vi "initialise.vi"(8 "error in (no error)":errorcluster, 11 "ScanHeadMH100729FPGA in":refnum<class "ScanHeadMH100729FPGA.lvclass">) -> (0 "error out":errorcluster, 3 "ScanHeadMH100729FPGA out":refnum<class "ScanHeadMH100729FPGA.lvclass">)   [LabVIEW 2010, in "ScanHeadMH100729FPGA.lvclass"]
uses:
  ScanHeadMH100729FPGA.lvclass
  GenericScanHead/GenericScanHead/GenericScanHead.lvclass
  ScanHeadMH100729FPGA.lvclass/ScanHeadMH100729FPGA.ctl
  AnalogOut/GenericAnalogOut/GenericAnalogOut/GenericAnalogOut.lvclass
  common/classes/ErrorController/ErrorController/class_data.vi
  common/classes/ErrorController/ErrorController/ErrorController.lvclass
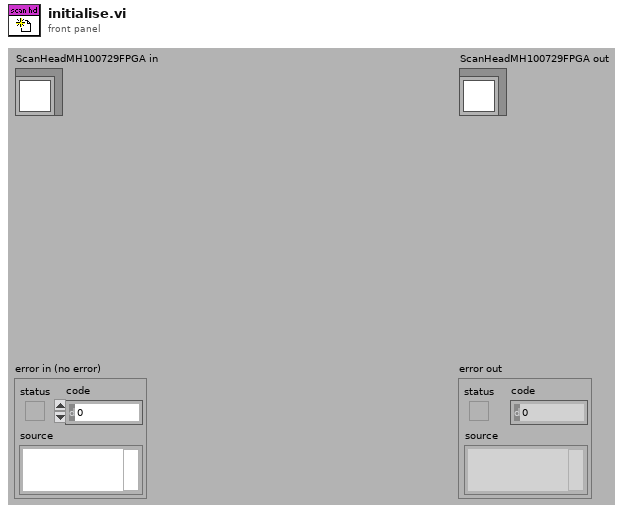
[diagram p1: front panel]
types:
  T1 = enum8{"Enabled", "Disabled", "Disabled and Grayed Out"}
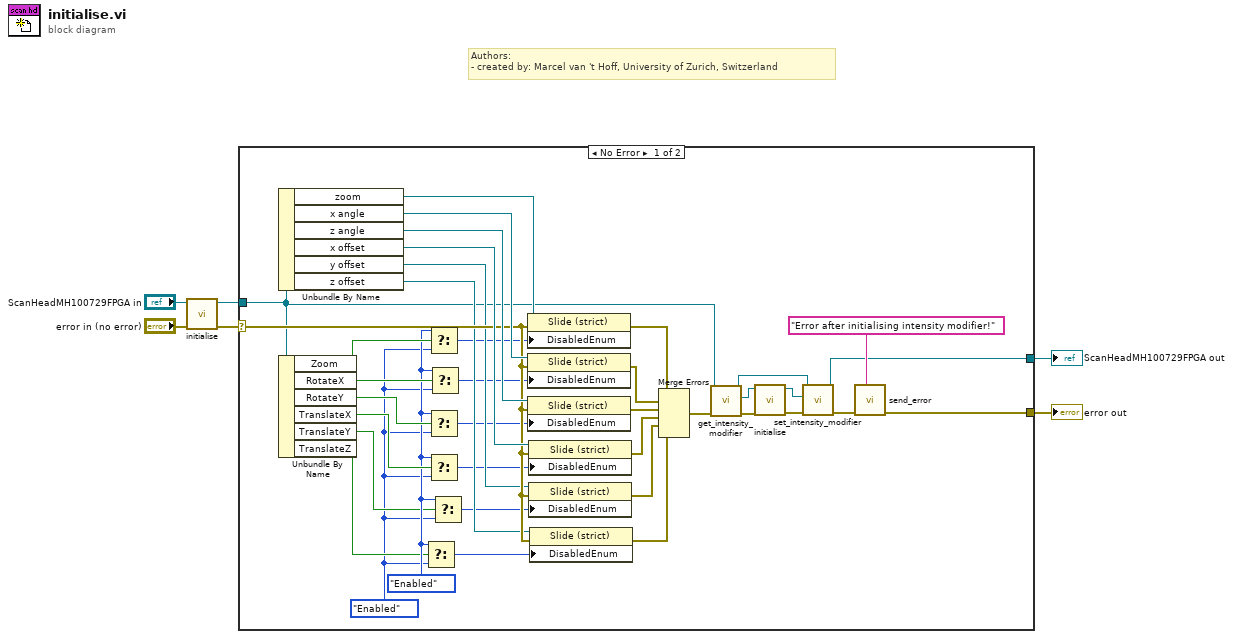
[diagram p0: block diagram]
diagram:
  # "Authors: \n- created by: Marcel van 't Hoff, University of Zurich, Switzerland"
  n1 = call-parent "initialise.vi"("error in (no error)"="error in (no error)", "GenericPlugin in"="ScanHeadMH100729FPGA in") -> ("error out"=w1:errorcluster, "GenericPlugin out"=w2:refnum<class "ScanHeadMH100729FPGA.lvclass">)  [unwired: 8 in]
  n2 = case shown="No Error" w1 {
    selector: w1 -> [w40 w45]
    tunnel: w2 -> [w10 w46]
    tunnel: [w7 w45] -> w6
    tunnel: [w8 w46] -> w5
    frame No Error {
      w19 = T1."Enabled" ("Disabled")
      w22 = T1."Enabled" ("Disabled")
      n3 = Unbundle By Name(w10) -> ("zoom"=w44:refnum<vi>, "x angle"=w43:refnum<vi>, "z angle"=w42:refnum<vi>, "x offset"=w41:refnum<vi>, "y offset"=w39:refnum<vi>, "z offset"=w38:refnum<vi>)
      n4 = Unbundle By Name(w10) -> ("Zoom"=w32:bool, "RotateX"=w31:bool, "RotateY"=w30:bool, "TranslateX"=w25:bool, "TranslateY"=w21:bool, "TranslateZ"=w20:bool)
      n5 = Select(t=w22, s=w20, f=w19) -> (s? t:f=w23:T1)
      n6 = Select(t=w22, s=w32, f=w19) -> (s? t:f=w29:T1)
      n7 = Select(t=w22, s=w30, f=w19) -> (s? t:f=w27:T1)
      n8 = Select(t=w22, s=w25, f=w19) -> (s? t:f=w26:T1)
      n9 = Select(t=w22, s=w31, f=w19) -> (s? t:f=w28:T1)
      n10 = Select(t=w22, s=w21, f=w19) -> (s? t:f=w24:T1)
      n11 = property class="Slide (strict)"(reference=w44, error in=w40, "DisabledEnum"=w29) -> (error out=w18:errorcluster)  [unwired: 1 out]
      n12 = property class="Slide (strict)"(reference=w43, error in=w40, "DisabledEnum"=w28) -> (error out=w37:errorcluster)  [unwired: 1 out]
      n13 = property class="Slide (strict)"(reference=w42, error in=w40, "DisabledEnum"=w27) -> (error out=w36:errorcluster)  [unwired: 1 out]
      n14 = property class="Slide (strict)"(reference=w41, error in=w40, "DisabledEnum"=w26) -> (error out=w35:errorcluster)  [unwired: 1 out]
      n15 = property class="Slide (strict)"(reference=w39, error in=w40, "DisabledEnum"=w24) -> (error out=w34:errorcluster)  [unwired: 1 out]
      n16 = property class="Slide (strict)"(reference=w38, error in=w40, "DisabledEnum"=w23) -> (error out=w33:errorcluster)  [unwired: 1 out]
      n17 = Merge Errors(w18, w37, w36, w35, w34, w33) -> (w16:errorcluster)
      n18 = call-dynamic "get_intensity_modifier.vi"("error in (no error)"=w16, "ScanHeadMH100729FPGA in"=w10) -> ("error out"=w15:errorcluster, "intensity modifier"=w14:refnum<class "GenericAnalogOut.lvclass">, "ScanHeadMH100729FPGA out"=w9:refnum<class "ScanHeadMH100729FPGA.lvclass">)  [unwired: 7 in]
      n19 = call-dynamic "initialise.vi"("error in (no error)"=w15, "GenericPlugin in"=w14) -> ("error out"=w13:errorcluster, "GenericPlugin out"=w11:refnum<class "GenericAnalogOut.lvclass">)  [unwired: 8 in]
      n20 = call-dynamic "set_intensity_modifier.vi"("error in (no error)"=w13, "intensity modifier"=w11, "ScanHeadMH100729FPGA in"=w9) -> ("error out"=w12:errorcluster, "ScanHeadMH100729FPGA out"=w8:refnum<class "ScanHeadMH100729FPGA.lvclass">)  [unwired: 7 in]
      n21 = call "send_error.vi"("additional message"="Error after initialising intensity modifier!", "error in (no error)"=w12) -> ("error out"=w7:errorcluster)  [unwired: 9 in]
    }
    frame Error {
    }
  }
  "error out" <- w6
  "ScanHeadMH100729FPGA out" <- w5
